vi "Create Cursor Lines.vi"(4 "Actual Range":T1, 5 "Cursor Line":T3, 7 "Cursor Position":T2, 8 "error in (no error)":errorcluster, 11 "Cursor Object In":refnum<vi>) -> (0 "error out":errorcluster, 3 "Cursor Object Out":refnum<vi>)   [LabVIEW 2020, in "3D Plot.lvclass"]
uses:
  3D Plot.lvclass
  Cursor Line.ctl
  Line Type.ctl
  Range Clusters.ctl
  NI_3D Picture Control.lvlib
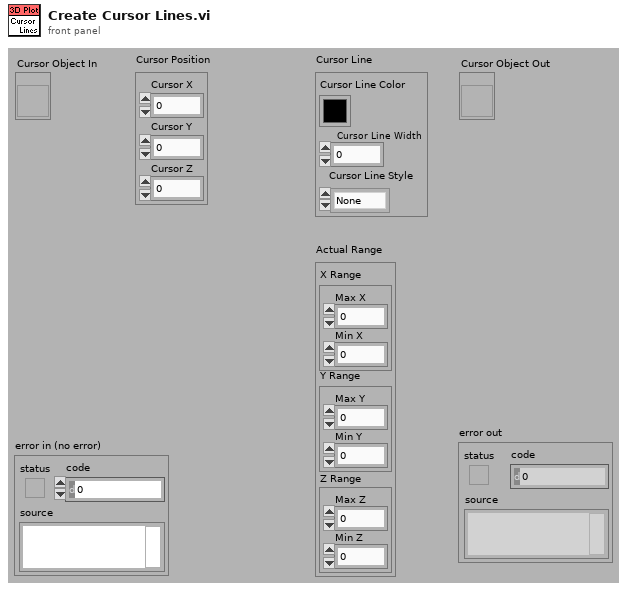
[diagram p1: front panel]
types:
  T1 = typedef "3D Plot.lvclass/Range Clusters.ctl" = cluster{"X Range":cluster{"Max X":sgl, "Min X":sgl}, "Y Range":cluster{"Max Y":sgl, "Min Y":sgl}, "Z Range":cluster{"Max Z":sgl, "Min Z":sgl}}
  T2 = cluster{"Cursor X":sgl, "Cursor Y":sgl, "Cursor Z":sgl}
  T3 = typedef "3D Plot.lvclass/Cursor Line.ctl" = cluster{"Cursor Line Color":u32, "Cursor Line Width":sgl, "Cursor Line Style":T4}
  T4 = typedef "3D Plot.lvclass/Line Type.ctl" = enum16{"None", "Solid", "Dash", "Dot", "Dash Dot"}
  T5 = enum16{"Normal Bin", "Opaque Bin", "Transparent Bin"}
  T6 = enum16{"Overall", "Per Primitive", "Per Vertex", "Binding Off"}
  T7 = enum16{"Points", "Lines", "Line Strip", "Line Loop", "Triangles", "Triangle Strip", "Triangle Fan", "Quads", "Quad Strip", "Polygon"}
  T8 = cluster{"Cursor X":sgl, "Cursor Y":sgl, "Cursor Z":sgl}[]
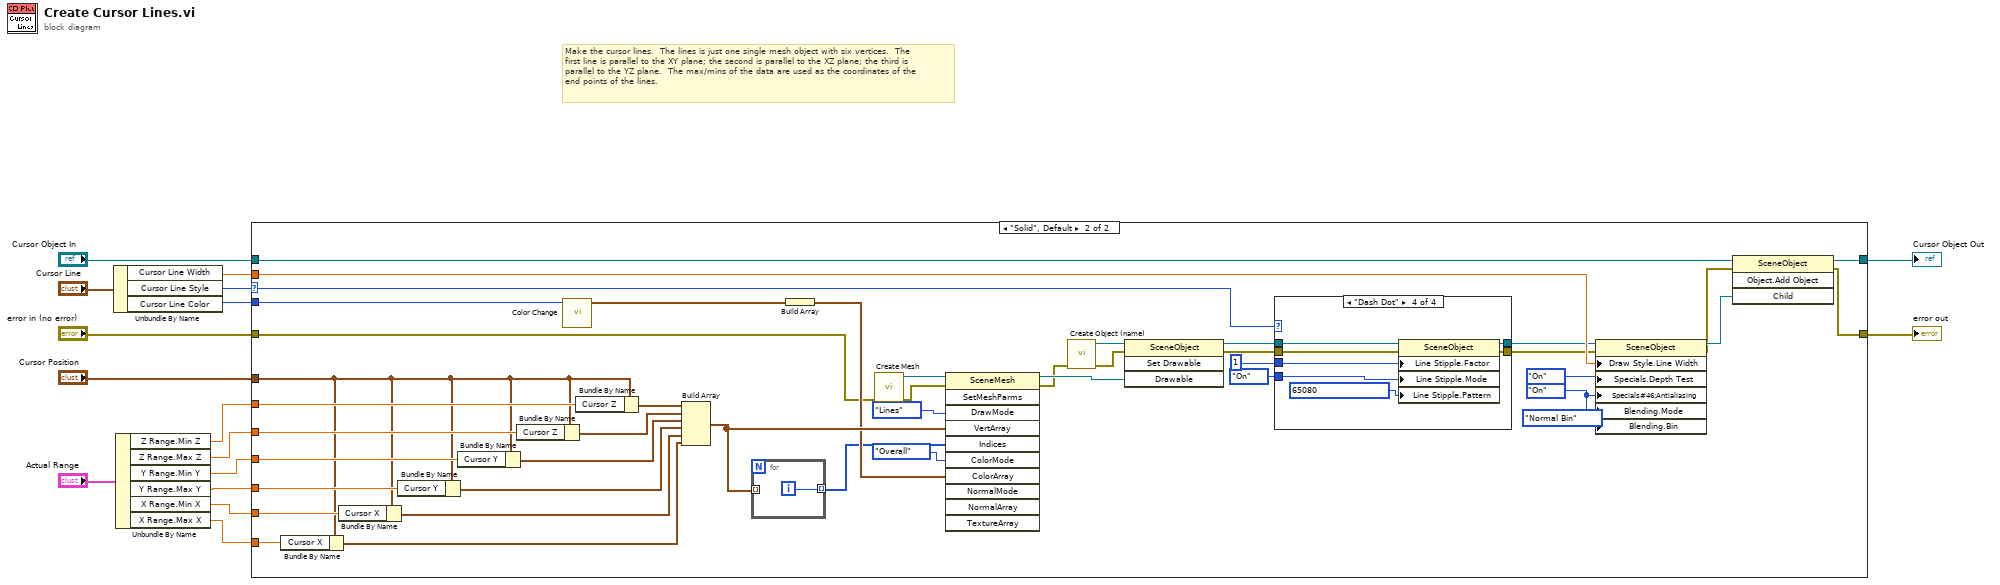
[diagram p0: block diagram]
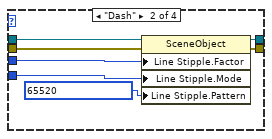
[diagram p4: hidden frame]
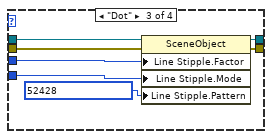
[diagram p5: hidden frame]
diagram:
  # "Make the cursor lines.  The lines is just one single mesh object with six vertices.  The first line is parallel to the XY plane; the second is parallel to the XZ plane; the third is parallel to the YZ plane.  The max/mins of the data are used as the coordinates of the end points of the lines."
  n1 = Unbundle By Name("Cursor Line") -> ("Cursor Line Width"=w2:sgl, "Cursor Line Style"=w10:T4, "Cursor Line Color"=w9:u32)
  n2 = Unbundle By Name("Actual Range") -> ("Z Range.Min Z"=w8:sgl, "Z Range.Max Z"=w7:sgl, "Y Range.Min Y"=w6:sgl, "Y Range.Max Y"=w5:sgl, "X Range.Min X"=w4:sgl, "X Range.Max X"=w3:sgl)
  n3 = case shown="\"Solid\", Default" w10 {
    selector: w10 -> [_ w19]
    tunnel: "Cursor Position" -> [_ w28]
    tunnel: "Cursor Object In" -> [w18 w45]
    tunnel: [w18 w44] -> w15
    tunnel: w7 -> [_ w58]
    tunnel: w9 -> [_ w48]
    tunnel: w2 -> [_ w43]
    tunnel: w8 -> [_ w40]
    tunnel: w6 -> [_ w39]
    tunnel: w5 -> [_ w38]
    tunnel: w4 -> [_ w37]
    tunnel: w3 -> [_ w36]
    tunnel: "error in (no error)" -> [w17 w34]
    tunnel: [w17 w29] -> w14
    frame "None" {
    }
    frame "Solid", Default {
      w26 = enum16{"Inherit Value", "Off", "On"}."On" ("Specials:Antialiasing")
      n4 = Bundle By Name(cluster=w28, "Cursor X"=w36) -> (w52:T2)
      n5 = Bundle By Name(cluster=w28, "Cursor X"=w37) -> (w53:T2)
      n6 = Bundle By Name(cluster=w28, "Cursor Y"=w38) -> (w54:T2)
      n7 = Bundle By Name(cluster=w28, "Cursor Y"=w39) -> (w55:T2)
      n8 = Bundle By Name(cluster=w28, "Cursor Z"=w58) -> (w56:T2)
      n9 = call "Color Change.vi"("Color"=w48) -> ("RGBA"=w47:cluster{"R":sgl, "G":sgl, "B":sgl, "A":sgl})  [unwired: 1 in, 9 out]
      n10 = Bundle By Name(cluster=w28, "Cursor Z"=w40) -> (w57:T2)
      n11 = Build Array(w57, w56, w55, w54, w53, w52) -> (w51:T8)
      n12 = for {
        tunnel: w51 -> [_] mode=indexing
        tunnel: [w85] -> w35 mode=indexing
        i -> [w85]
      }
      n13 = Build Array(w47) -> (w46:cluster{"R":sgl, "G":sgl, "B":sgl, "A":sgl}[])
      n14 = call "Create Mesh.vi"("error in (no error)"=w34) -> ("error out"=w33:errorcluster, "New Mesh Refnum"=w60:refnum<vi>)  [unwired: 9 out]
      n15 = invoke class="SceneMesh" method="SetMeshParms"(reference=w60, error in=w33, "DrawMode"=T7."Lines" ("Draw Mode"), "VertArray"=w51, "Indices"=w35, "ColorMode"=T6."Overall" ("Color Binding Mode"), "ColorArray"=w46) -> (reference out=w59:refnum<vi>, error out=w32:errorcluster)  [unwired: 4 in, 9 out]
      n16 = call "Create Object (name).vi"("error in (no error)"=w32) -> ("error out"=w31:errorcluster, "Scene:New Object"=w61:refnum<vi>)  [unwired: 9 in]
      n17 = invoke class="SceneObject" method="Set Drawable"(reference=w61, error in=w31, "Drawable"=w59) -> (reference out=w23:refnum<vi>, error out=w22:errorcluster)  [unwired: 1 in, 2 out]
      n18 = case shown="\"Dash Dot\"" w19 {
        tunnel: w23 -> [w63 w70 w77 w84]
        tunnel: [w63 w69 w73 w80] -> w21
        tunnel: w22 -> [w62 w68 w76 w83]
        tunnel: [w62 w67 w72 w79] -> w20
        tunnel: enum16{"Inherit Value", "Off", "On"}."On" ("Line Stipple:Mode") -> [_ w66 w74 w81]
        tunnel: 1 ("Line Stipple:Factor") -> [_ w65 w75 w82]
        frame "Solid", Default {
        }
        frame "Dash" {
          n19 = property class="SceneObject"(reference=w70, error in=w68, "Line Stipple.Factor"=w65, "Line Stipple.Mode"=w66, "Line Stipple.Pattern"=u16 65520 ("Line Stipple:Factor")) -> (reference out=w69:refnum<vi>, error out=w67:errorcluster)
        }
        frame "Dot" {
          n20 = property class="SceneObject"(reference=w77, error in=w76, "Line Stipple.Factor"=w75, "Line Stipple.Mode"=w74, "Line Stipple.Pattern"=u16 52428 ("Line Stipple:Factor")) -> (reference out=w73:refnum<vi>, error out=w72:errorcluster)
        }
        frame "Dash Dot" {
          n21 = property class="SceneObject"(reference=w84, error in=w83, "Line Stipple.Factor"=w82, "Line Stipple.Mode"=w81, "Line Stipple.Pattern"=u16 65080 ("Line Stipple:Factor")) -> (reference out=w80:refnum<vi>, error out=w79:errorcluster)
        }
      }
      n22 = property class="SceneObject"(reference=w21, error in=w20, "Draw Style.Line Width"=w43, "Specials.Depth Test"=enum16{"Inherit Value", "Off", "On"}."On" ("Specials:Depth Test"), "Specials#46;Antialiasing"=w26, "Blending.Mode"=w26, "Blending.Bin"=T5."Normal Bin" ("Blending:Bin")) -> (reference out=w41:refnum<vi>, error out=w30:errorcluster)
      n23 = invoke class="SceneObject" method="Object.Add Object"(reference=w45, error in=w30, "Child"=w41) -> (reference out=w44:refnum<vi>, error out=w29:errorcluster)  [unwired: 1 in, 2 out]
    }
  }
  "Cursor Object Out" <- w15
  "error out" <- w14
